vi "SelectMenu.vi"(0 "XRef":T10, 1 "Tag":T6, 2 "Point":T8, 3 "Click Type":T7, 4 "State In":T1 {"BlockNodeState"."Draw Style" items=["FunctionBlock", "ExpressVI", "Variable", "Elemental I/O", "32x32 Icon", "FunctionBlockCompact"]; "BlockNodeState"."Terminal Data"."Terminal Flags" format="%.0b"}) -> (14 "Reply":T5, 16 "State Out":T1 {"BlockNodeState"."Draw Style" items=["FunctionBlock", "ExpressVI", "Variable", "Elemental I/O", "32x32 Icon", "FunctionBlockCompact"]; "BlockNodeState"."Terminal Data"."Terminal Flags" format="%.0b"})   [LabVIEW 2020, in "Digital_Group.xnode"]
uses:
  <vilib>/express/express signal manip/DigitalDataGroupingXNode/Digital_Group.xnode
  <vilib>/XNodeSupport/XNodeXNodeRef.ctl
  <vilib>/XNodeSupport/XNodeString.ctl
  <vilib>/XNodeSupport/XNodePoint.ctl
  <vilib>/XNodeSupport/XNodeInt.ctl
  <vilib>/XNodeSupport/XNodeClickTypes.ctl
  <vilib>/express/express signal manip/DigitalDataGroupingXNode/State.ctl
  <vilib>/BlockNodeSupport/TerminalData.ctl
  <vilib>/picture/picture.llb/imagedata.ctl
  <vilib>/express/express signal manip/DigitalDataGroupingXNode/DigitalGroup_Recording Cluster.ctl
  <vilib>/XNodeSupport/XNodeStringArray.ctl
  <vilib>/XNodeSupport/NI_XNodeSupport.lvlib
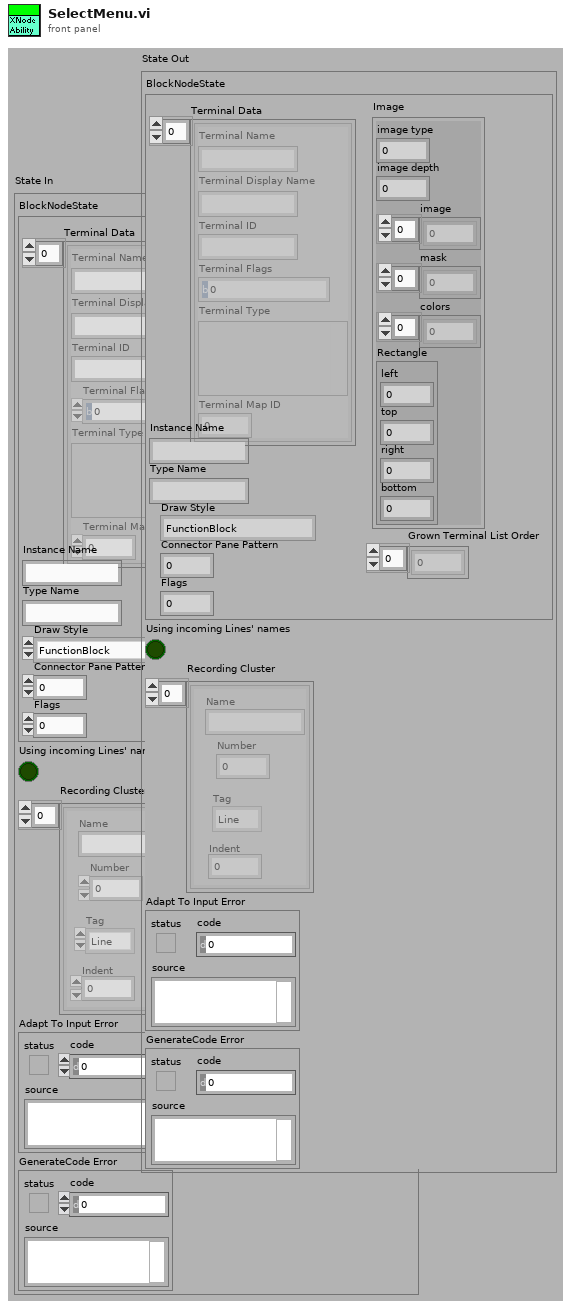
[diagram p1: front panel]
types:
  T1 = typedef "Digital_Group.xnode/State.ctl" = cluster{"BlockNodeState":cluster{"Terminal Data":T2[], "Instance Name":string, "Type Name":string, "Draw Style":i32, "Connector Pane Pattern":i32, "Flags":i32, "Grown Terminal List Order":i32[], "Image":T3}, "Using incoming Lines' names":bool, "Recording Cluster":T4, "Adapt To Input Error":errorcluster, "GenerateCode Error":errorcluster}
  T2 = typedef "TerminalData.ctl" = cluster{"Terminal Name":string, "Terminal Display Name":string, "Terminal ID":string, "Terminal Flags":i32, "Terminal Type":variant, "Terminal Map ID":i32}
  T3 = typedef "imagedata.ctl" = cluster{"image type":i32, "image depth":i32, "image":u8[], "mask":u8[], "colors":u32[], "Rectangle":cluster{"left":i16, "top":i16, "right":i16, "bottom":i16}}
  T4 = typedef "DigitalGroup_Recording Cluster.ctl" = cluster{"Name":string, "Number":u32, "Indent":u32, "Tag":enum16{"Line", "Opened Bus", "Closed Bus"}}[]
  T5 = typedef "NI_XNodeSupport.lvlib/XNodeStringArray.ctl" = T6[]
  T6 = typedef "NI_XNodeSupport.lvlib/XNodeString.ctl" = string
  T7 = typedef "NI_XNodeSupport.lvlib/XNodeClickTypes.ctl" = enum32{"Operate Click", "Popup Click"}
  T8 = typedef "NI_XNodeSupport.lvlib/XNodePoint.ctl" = cluster{"H":T9, "V":T9}
  T9 = typedef "NI_XNodeSupport.lvlib/XNodeInt.ctl" = i32
  T10 = typedef "NI_XNodeSupport.lvlib/XNodeXNodeRef.ctl" = refnum<vi>
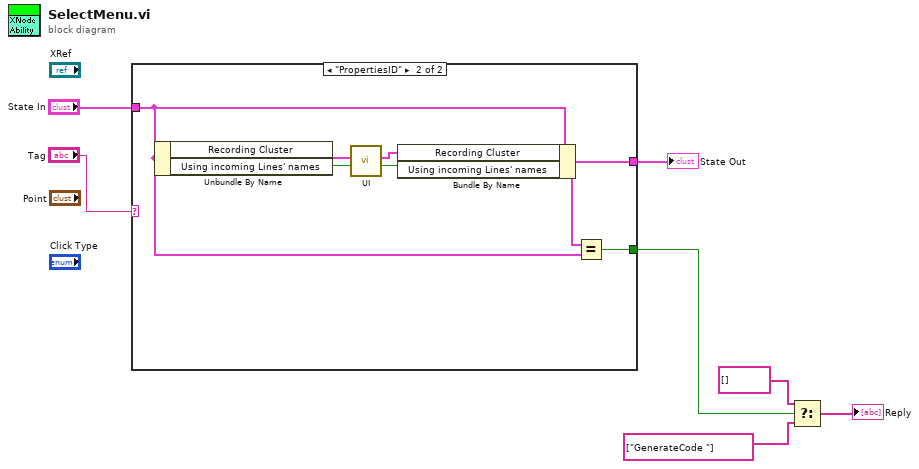
[diagram p0: block diagram]
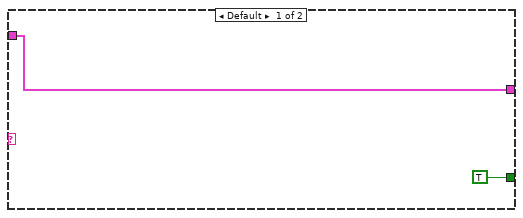
[diagram p2: hidden frame]
diagram:
  n1 = case shown="\"PropertiesID\"" "Tag" {
    tunnel: "State In" -> [w9 w11]
    tunnel: [w9 w12] -> w6
    tunnel: [TRUE w10] -> w1
    frame Default {
    }
    frame "PropertiesID" {
      n2 = Unbundle By Name(w11) -> ("Recording Cluster"=w16:T4, "Using incoming Lines' names"=w15:bool)
      n3 = call <vilib>:"UI.vi"("Use incoming waveform names"=w15, "In Recording Cluster"=w16) -> ("Use Incoming Waveform Names 2"=w13:bool, "Recording Cluster"=w14:T4)  [unwired: 7 in, 1 out]
      n4 = Bundle By Name(cluster=w11, "Recording Cluster"=w14, "Using incoming Lines' names"=w13) -> (w12:T1)
      n5 = Equal?(x=w12, y=w11) -> (x = y?=w10:bool)
    }
  }
  "State Out" <- w6
  n6 = Select(t=T5 [] ("f"), s=w1, f=T5 ["GenerateCode "] ("Reply")) -> (s? t:f=→"Reply":T5)
